vi "Add Terminals.vi"(6 "acyclic frame names":string[](array[string]), 8 "error in":errorcluster, 9 "terminal names":string[](array[string]), 10 "terminal addresses":T2[](array[typedef]), 11 "port":T1 format="%.0x") -> (0 "error out":errorcluster, 3 "port out":T1 format="%.0x")   [LabVIEW 2020, in "AIM MIL-STD-1553 Scripting.lvlib"]
doc: "Iterates through the <b>terminal addresses</b> array and the <b>terminal names</b> provided and adds the terminals to the <b>port</b>. If a Terminal Address is 0, the Terminal is named \"Bus Controller\" and added as the Bus Controller, otherwise it is added as a Remote Terminal.\n\nIf a Bus Controller is added, the <b>acyclic frame names</b> will be added to the Acyclic Frames Section of the Bus Controller"
uses:
  AIM MIL-STD-1553 Scripting.lvlib
  Shared/Address.ctl
  <vilib>/NI VeriStand/Custom Device API/Custom Device Item Ref.ctl
  <vilib>/NI VeriStand/Custom Device API/Custom Device API.lvlib
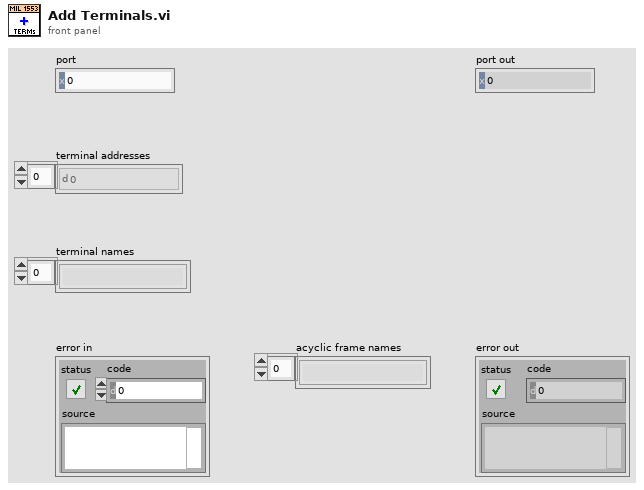
[diagram p1: front panel]
types:
  T1 = typedef "Custom Device API.lvlib/Custom Device Item Ref.ctl" = u64
  T2 = typedef "Address.ctl" = u16
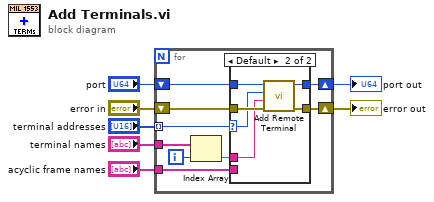
[diagram p0: block diagram]
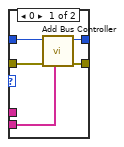
[diagram p2: hidden frame]
diagram:
  n1 = for {
    shift-right: [w13] -> w3
    shift-left: "error in" -> [w14]
    tunnel: "terminal addresses" -> [w16] mode=indexing
    tunnel: "acyclic frame names" -> [w12]
    shift-right: [w11] -> w4
    shift-left: "port" -> [w15]
    tunnel: "terminal names" -> [w9]
    i -> [w8]
    n2 = Index Array(array=w9, index=w8) -> (element=w10:string)
    n3 = case shown="Default" w16 {
      selector: w16 -> [_ w24]
      tunnel: w15 -> [w21 w25]
      tunnel: w14 -> [w20 w27]
      tunnel: [w19 w26] -> w13
      tunnel: w12 -> [w17 _]
      tunnel: [w18 w23] -> w11
      tunnel: w10 -> [_ w22]
      frame 0 {
        n4 = call "Add Bus Controller.vi"("acyclic frame names"=w17, "error in"=w20, "port"=w21) -> ("error out"=w19:errorcluster, "port out"=w18:T1)  [unwired: 6 in, 1 out]
      }
      frame Default {
        n5 = call "Add Remote Terminal.vi"("error in"=w27, "terminal name"=w22, "terminal address"=w24, "port"=w25) -> ("error out"=w26:errorcluster, "port out"=w23:T1)  [unwired: 5 in, 1 out]
      }
    }
  }
  "port out" <- w4
  "error out" <- w3
